vi "SanitizePathComponents.vi"(1 "PathComponentsIn":string[](array[string])) -> (0 "SanitizedComponentsOut":string[](array[string]))   [LabVIEW 2015]
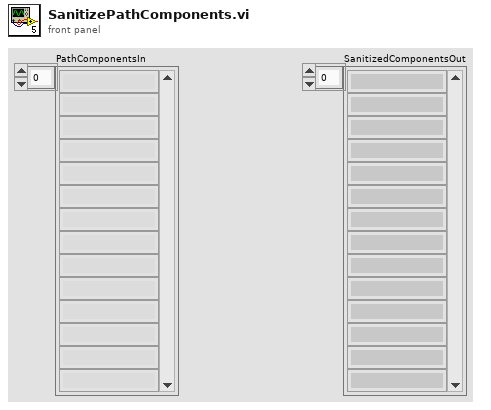
[diagram p1: front panel]
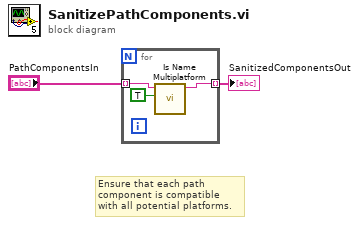
[diagram p0: block diagram]
diagram:
  # "Ensure that each path\ncomponent is compatible\nwith all potential platforms."
  n1 = for {
    tunnel: [w5] -> w1 mode=indexing
    tunnel: "PathComponentsIn" -> [w3] mode=indexing
    n2 = call <vilib>:"Is Name Multiplatform.vi"("name must work for all platforms (F)"=TRUE, "filename"=w3) -> ("suggested filename"=w5:string)  [unwired: 5 in, 4 out]
  }
  "SanitizedComponentsOut" <- w1
